vi "FTW-Endpoint-TCP-Reply-Worker.vi"(0 "TCP Endpoint":refnum<class "FTW-Endpoint-TCP.lvclass">) -> ()   [LabVIEW 2013, in "FTW-Endpoint-TCP.lvclass"]
uses:
  FTW-Endpoint-TCP.lvclass
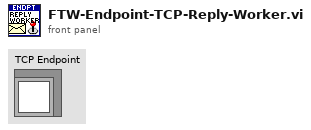
[diagram p1: front panel]
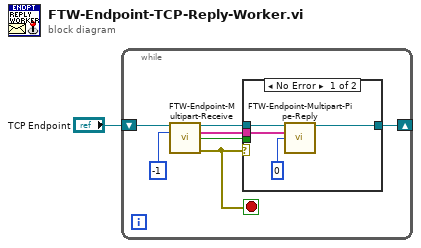
[diagram p0: block diagram]
diagram:
  n1 = while {
    shift-right: [w8] -> _
    shift-left: "TCP Endpoint" -> [w7]
    stop <- w2 stop-if-true
    n2 = call-dynamic "FTW-Endpoint-Multipart-Receive.vi"("FTW Endpoint"=w7, "Timeout"=-1) -> ("FTW Endpoint out"=w6:refnum<class "FTW-Endpoint-TCP.lvclass">, "Message Received"=w3:string[], "Timed out?"=w4:bool, "error out"=w2:errorcluster)  [unwired: 10 in]
    n3 = case shown="No Error" w2 {
      tunnel: [w12 w13] -> w8
      tunnel: w6 -> [w11 w13]
      tunnel: w4 -> [_ _]
      tunnel: w3 -> [w10 _]
      frame No Error {
        n4 = call-dynamic "FTW-Endpoint-Multipart-Pipe-Reply.vi"("FTW Endpoint"=w11, "Multipart Message"=w10, "Timeout"=0) -> ("FTW Endpoint out"=w12:refnum<class "FTW-Endpoint-TCP.lvclass">)  [unwired: 10 in, 2 out]
      }
      frame Error {
      }
    }
  }
